vi "Parralel Proportional Calculation.vi"(9 "FeedFwd Amount":dbl format="%.2f", 10 "PID gains":T1, 11 "Error":dbl) -> (3 "Proportional Term":dbl)   [LabVIEW 2020]
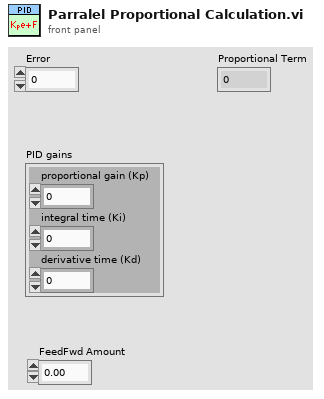
[diagram p1: front panel]
types:
  T1 = cluster{"proportional gain (Kp)":dbl, "integral time (Ki)":dbl, "derivative time (Kd)":dbl}
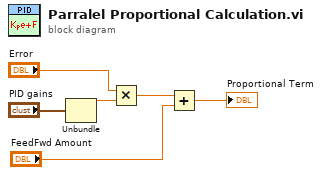
[diagram p0: block diagram]
diagram:
  n1 = Unbundle("PID gains") -> ("proportional gain (Kp)"=w6:dbl)  [unwired: 2 out]
  n2 = Multiply(x="Error", y=w6) -> (x*y=w3:dbl)
  n3 = Add(x=w3, y="FeedFwd Amount") -> (x+y=→"Proportional Term":dbl)
